vi "Reorder Page TOC.vi"(0 "PDF Report IN":refnum<class "PDF Report Class.lvclass">, 5 "Number pages after TOC":i32, 7 "Number pages before TOC":i32, 9 "TOC start at page":i32, 11 "error in (no error)":errorcluster) -> (4 "PDF Report OUT":refnum<class "PDF Report Class.lvclass">, 8 "Pages [ ]":i32[](array[numeric]), 15 "error out":errorcluster)   [LabVIEW 2019, in "Exaprom PDF.lvlib"]
doc: "Version 1.1\nDeveloped by Jean-Marc Simard\nCopyright © 2012, Exaprom Inc.\nAll rights reserved.\nLicense: BSD\n\nWith iTextSharp 4.1.6 (http://itextsharp.sourceforge.net)\nunder Mozilla Public License Version 1.1\n(http://www.mozilla.org/MPL/MPL-1.1.html)"
uses:
  LV Class/PDF Report Class/PDF Report Class.lvclass
  Exaprom PDF.lvlib
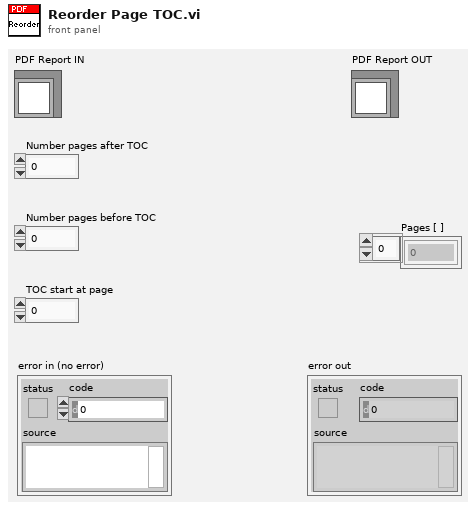
[diagram p1: front panel]
types:
  T1 = typedef "Exaprom PDF.lvlib/Page dimensions.ctl" = cluster{"Start at page":i32, "Page Size":T2, "Orientation":T3, "widht":sgl, "height":sgl, "Margin left":sgl, "Margin right":sgl, "Margin top":sgl, "Margin bottom":sgl, "X0":sgl, "X1":sgl, "Y0":sgl, "Y1":sgl}
  T2 = typedef "Exaprom PDF.lvlib/Page size.ctl" = i32
  T3 = typedef "Exaprom PDF.lvlib/Page Orientation.ctl" = enum16{"Portrait", "Landscape"}
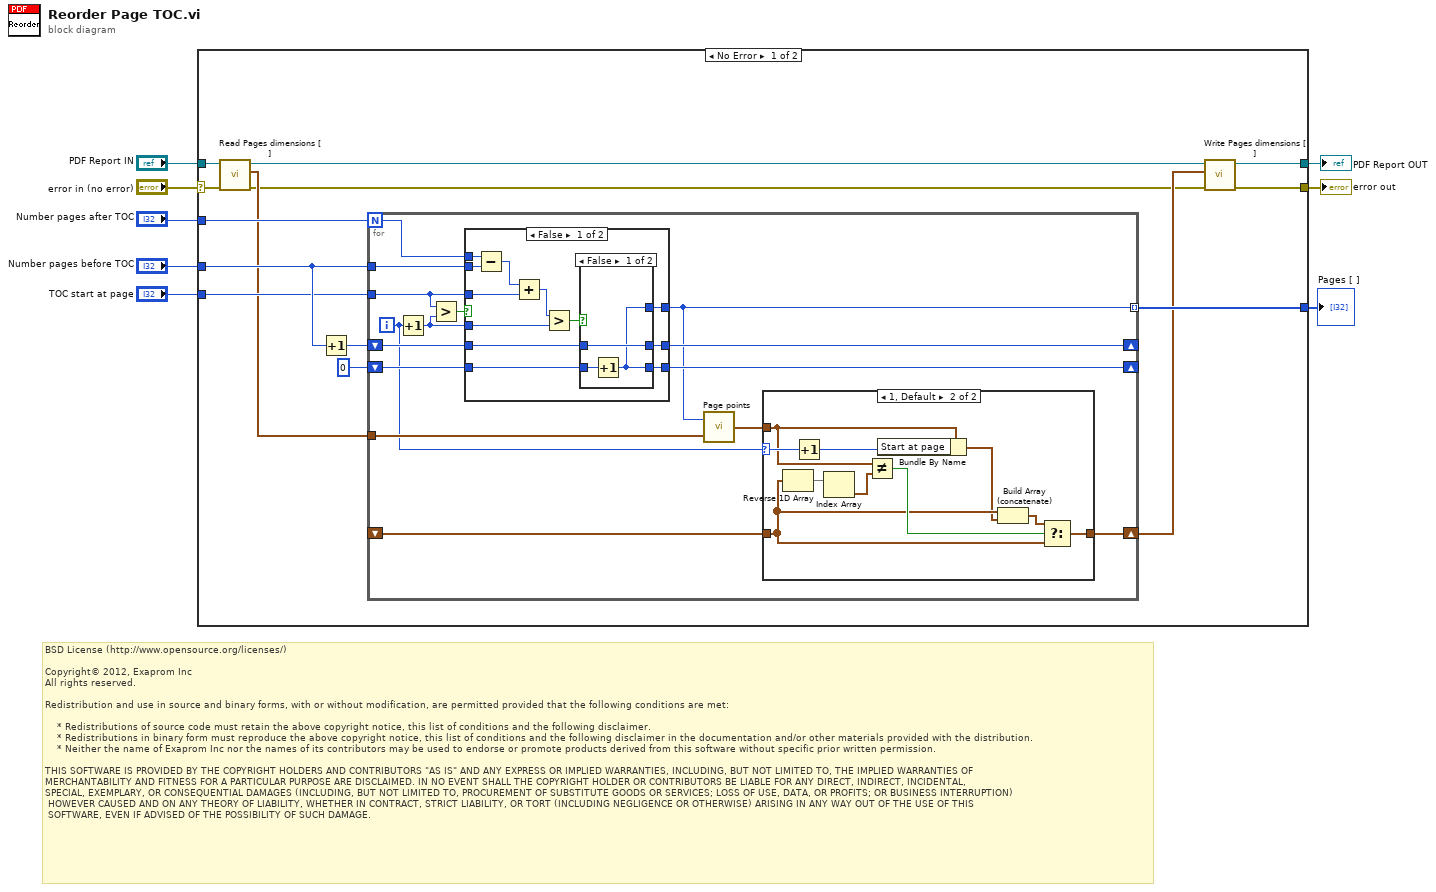
[diagram p0: block diagram]
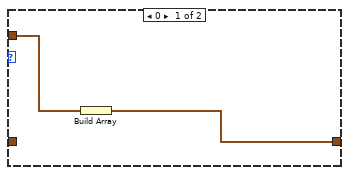
[diagram p2: hidden frame]
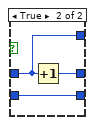
[diagram p3: hidden frame]
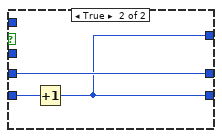
[diagram p4: hidden frame]
diagram:
  # "BSD License (http://www.opensource.org/licenses/)\n\nCopyright© 2012, Exaprom Inc\nAll rights reserved.\n\nRedistribution and use in source and binary forms, with or without modification, are permitted provided that the following conditions are met:\n\n    * Redistributions of source code must retain the above copyright notice, this list of conditions and the following disclaimer.\n    * Redistributions in binary form must reproduce the above copyright notice, this list of conditions and the following disclaimer in the documentation and/or other materials provided with the distribution.\n    * Neither the name of Exaprom Inc nor the names of its contributors may be used to endorse or promote products derived from this software without specific prior written permission.\n\nTHIS SOFTWARE IS PROVIDED BY THE COPYRIGHT HOLDERS AND CONTRIBUTORS \"AS IS\" AND ANY EXPRESS OR IMPLIED WARRANTIES, INCLUDING, BUT NOT LIMITED TO, THE IMPLIED WARRANTIES OF \nMERCHANTABILITY AND FITNESS FOR A PARTICULAR PURPOSE ARE DISCLAIMED. IN NO EVENT SHALL THE COPYRIGHT HOLDER OR CONTRIBUTORS BE LIABLE FOR ANY DIRECT, INDIRECT, INCIDENTAL,\nSPECIAL, EXEMPLARY, OR CONSEQUENTIAL DAMAGES (INCLUDING, BUT NOT LIMITED TO, PROCUREMENT OF SUBSTITUTE GOODS OR SERVICES; LOSS OF USE, DATA, OR PROFITS; OR BUSINESS INTERRUPTION)\n HOWEVER CAUSED AND ON ANY THEORY OF LIABILITY, WHETHER IN CONTRACT, STRICT LIABILITY, OR TORT (INCLUDING NEGLIGENCE OR OTHERWISE) ARISING IN ANY WAY OUT OF THE USE OF THIS\n SOFTWARE, EVEN IF ADVISED OF THE POSSIBILITY OF SUCH DAMAGE."
  n1 = case shown="No Error" "error in (no error)" {
    selector: "error in (no error)" -> [w15 w72]
    tunnel: "PDF Report IN" -> [w22 w71]
    tunnel: [w12 w71] -> w7
    tunnel: [w10 w72] -> w6
    tunnel: "Number pages after TOC" -> [w19 _]
    tunnel: "Number pages before TOC" -> [w18 _]
    tunnel: "TOC start at page" -> [w17 _]
    tunnel: [w13 _] -> w1
    frame No Error {
      n2 = call-dynamic "Read Pages dimensions [ ].vi"("error in (no error)"=w15, "PDF Report Class in"=w22) -> ("error out"=w9:errorcluster, "Pages dimensions [ ]"=w14:T1[], "PDF Report Class out"=w16:refnum<class "PDF Report Class.lvclass">)  [unwired: 6 in, 1 out]
      n3 = Increment(x=w18) -> (x+1=w20:i32)
      n4 = for {
        N: w19 -> [w34]
        tunnel: w17 -> [w35]
        tunnel: [w27] -> w13 mode=indexing
        tunnel: w18 -> [w36]
        shift-right: [w33] -> _
        shift-left: w20 -> [w32]
        shift-right: [w30] -> _
        shift-left: 0 -> [w31]
        shift-right: [w24] -> w11
        shift-left: _ -> [w25]
        tunnel: w14 -> [w29]
        i -> [w26]
        n5 = Increment(x=w26) -> (x+1=w28:i32)
        n6 = Greater?(x=w35, y=w28) -> (0:w37:bool)
        n7 = case shown="False" w37 {
          tunnel: [w61 w68] -> w27
          tunnel: w28 -> [w53 _]
          tunnel: w36 -> [w58 _]
          tunnel: w35 -> [w55 _]
          tunnel: w34 -> [w57 _]
          tunnel: [w59 w70] -> w33
          tunnel: w32 -> [w60 w70]
          tunnel: w31 -> [w51 w69]
          tunnel: [w50 w68] -> w30
          frame False {
            n8 = Subtract(x=w57, y=w58) -> (x-y=w56:i32)
            n9 = Add(x=w56, y=w55) -> (x+y=w54:i32)
            n10 = Greater?(x=w54, y=w53) -> (0:w52:bool)
            n11 = case shown="False" w52 {
              tunnel: [w62 w67] -> w61
              tunnel: w60 -> [w64 w67]
              tunnel: [w64 w66] -> w59
              tunnel: w51 -> [w63 w65]
              tunnel: [w62 w65] -> w50
              frame False {
                n12 = Increment(x=w63) -> (x+1=w62:i32)
              }
              frame True {
                n13 = Increment(x=w67) -> (x+1=w66:i32)
              }
            }
          }
          frame True {
            n14 = Increment(x=w69) -> (x+1=w68:i32)
          }
        }
        n15 = call "Page points.vi"("Pages dimensions [ ]"=w29, "pageNum"=w27) -> ("Page (points)"=w23:T1)
        n16 = case shown="1, Default" w26 {
          selector: w26 -> [_ w43]
          tunnel: w25 -> [_ w45]
          tunnel: [w39 w47] -> w24
          tunnel: w23 -> [w38 w41]
          frame 0 {
            n17 = Build Array(w38) -> (w39:T1[])
          }
          frame 1, Default {
            n18 = Reverse 1D Array(array=w45) -> (reversed array=w49:T1[])
            n19 = Increment(x=w43) -> (x+1=w42:i32)
            n20 = Index Array(array=w49) -> (element=w48:T1)  [unwired: 1 in]
            n21 = Not Equal?(x=w41, y=w48) -> (x != y?=w46:bool)
            n22 = Bundle By Name(cluster=w41, "Start at page"=w42) -> (w40:T1)
            n23 = Build Array (concatenate)(w45, w40) -> (w44:T1[])
            n24 = Select(t=w44, s=w46, f=w45) -> (s? t:f=w47:T1[])
          }
        }
      }
      n25 = call-dynamic "Write Pages dimensions [ ].vi"("error in (no error)"=w9, "Pages dimensions [ ]"=w11, "PDF Report Class in"=w16) -> ("error out"=w10:errorcluster, "PDF Report Class out"=w12:refnum<class "PDF Report Class.lvclass">)  [unwired: 7 in]
    }
    frame Error {
    }
  }
  "PDF Report OUT" <- w7
  "error out" <- w6
  "Pages [ ]" <- w1
